vi "Scan and Trace(Unfold Normal Speed).vi"() -> ()   [LabVIEW 2020]
uses:
  Labview Library/Libraries/Basic Experiment/Basic Experiment.lvlib
  Labview Library/Libraries/LaoJi/NI CTR/NI DAQ Counter.lvlib
  Labview Library/Libraries/PIScanner_new/Library/PIScanner.lvlib
panel:
  in  "Stop Scan":bool
  in  "Stop ALL":bool=TRUE
  out "Laser On":bool
  out "Current Position":dbl[](array[numeric])=[149.3013306, 92.52485657, 114.2977448]
  in  "Tab Control":T1(tab)
  in  "md File Path":path=path "I:/Important Scan Image/Find SIV.md"
  in  "Comment":string="下午重新写了ASG的程序，把之前的Laser什么的用新的程序改掉了，然后把程序里面的计数都用老季的改掉了"
  in  "Title":string="扫描XZ"
  in  "Scan Parameter":T2={"horizontal start"=10.0, "horizontal end"=190.0, "horizontal num"=40, "vertical start"=100.0, "vertical end"=160.0, "vertical num"=40}
  out "Intensity Graph":dbl[][](graph)=[[17781.40531401807, 5714.199786500514, 6283.714545371459, 6735.417820419619, 5516.371803474795, 7255.943323026121, 6467.242901396061, 11976.047904166111, 11638.851498312759, 33572.80368126317, 34644.84074795653, 11401.592204703611, 12777.968493765737, 16629.229580655952, 14525.548166527793, 26871.089749350882, 27700.971050532404, 26252.009210884047, 25345.291111593357, 22513.920437453515, 23987.33624029484, 23198.350772809936, 23001.433789688253, 23079.35827112529, 24582.896751616194, 22567.526269993323, 24264.76234359153, 22164.571946750242, 25398.356910744176, 21846.320324133354, 22342.246318034588, 24552.890412679728, 24617.940704268913, 21673.961690578664, 26341.4103776154, 23416.335588634272, 24165.213215005195, 21944.877795249304, 24289.577304311242, 23535.77278446977, 25519.2278536345], [12532.419773169353, 6756.365461451473, 5205.122244571681, 6640.994524713253, 5430.964469504035, 7784.6001147647185, 6877.126979041758, 12219.704514135643, 12149.51945578161, 31845.833503515085, 35459.51140053275, 12611.918262761195, 10461.664756189162, 15261.448655811466, 13971.079864781508, 29604.672953223595, 26585.433397884048, 26165.899763849535, 22610.420936584742, 24458.55473918764, 21202.20584482011, 22676.314716648474, 22852.49041256598, 21138.005322471614, 23202.639601690946, 23660.949017499315, 22138.91430764288, 23771.110418104054, 22131.508001735023, 23840.890321990857, 22513.23380272118, 22045.969737474737, 22009.927882442946, 26290.801792700036, 22550.881393922507, 23976.253997987915, 23209.151892740247, 21374.168364274912, 22886.1538768692, 22109.997236054605, 22247.049582562136], [11023.148612036859, 6069.880132632881, 6091.825744562944, 6785.714285685821, 6272.541947646212, 7394.588598920568, 6863.383847160945, 12491.059826098322, 11518.116836241139, 33022.96459391927, 32198.322866861687, 12239.159240629258, 10380.206400641651, 15867.913649992137, 15146.431954406176, 29088.75642993861, 28241.281926540338, 25375.18296954822, 24239.543726400287, 22402.275786833994, 23427.467970935504, 19542.00015163378, 22868.559027272375, 23480.382191633205, 20472.903807809227, 23607.132086915753, 22000.15103086426, 21024.698918047514, 23190.641721682656, 21132.816105685317, 23244.46434584329, 20836.027647314855, 20762.358720963322, 24523.97567534188, 23514.537347734593, 22355.4414949403, 22273.56939147543, 22333.351986807338, 21172.97292010603, 23223.122196765806, 24603.867748041343], [12734.597431764863, 6547.24759851939, 6416.618185537506, 5721.2403649376465, 5517.269052163687, 6015.6693864512035, 6753.645433656194, 12558.695509637037, 10756.152568869344, 31460.58872169549, 29049.138481258386, 11605.03335797576, 12437.873324350952, 17971.080543714357, 17242.00048384432, 28463.531419469364, 27475.425557442424, 26130.076311780726, 23883.4365556246, 23337.802274226877, 23996.129656380228, 22192.4179121422, 22839.91858432976, 21200.737241837916, 20902.390142804205, 24376.990912244193, 20471.9645018656, 24101.790691422255, 20445.865161215617, 22588.842725292176, 21766.153377964467, 24164.48230671008, 21458.55170514228, 24138.01737736392, 24437.465471435327, 22589.395355642413, 21022.36718033937, 23901.075548187724, 21333.252640294686, 23447.659501746144, 21647.470177122526], [13703.182922298633, 5847.981715258857, 6706.874546456047, 6398.55097428461, 6057.052589773717, 6495.037310448332, 7086.934661307756, 13978.25044774562, 13984.747570265346, 34137.82564325823, 32511.9610057858, 13027.2184658737, 13741.34295395774, 17104.746207888747, 17614.610856088933, 28716.700446135794, 25474.792952360327, 25993.334782884132, 26240.48163660691, 22965.466183809942, 23424.85447434729, 24130.717249332658, 23824.887079750475, 21671.91895887727, 21540.144773083164, 22493.36115814037, 21465.475127230937, 21198.15668224017, 22004.76852760417, 23441.069548457646, 22470.987800033847, 22425.468296537474, 22085.716729267533, 21966.897808341815, 21877.303983712707, 22933.978416931946, 21511.349004124007, 23042.548454102853, 23403.759476785068, 23031.02748277378, 21486.356423589263], [12946.458625764166, 5592.979573231455, 5355.55804911163, 6146.06995703598, 5811.338679804044, 6541.940535257157, 7146.4081531214715, 15118.615175448802, 14260.249554349572, 38472.66562819246, 28917.599545080768, 14560.161779681965, 11942.44038600165, 16361.727963159978, 16676.65922683603, 25432.611286917556, 27901.729504499723, 23724.058258230565, 24343.84948213968, 20859.21325040204, 22430.7095897709, 23433.51497685545, 22768.02231275929, 22997.335154221877, 22810.76548338465, 22314.50442798871, 24192.1060310366, 21689.561203437006, 24769.464919970418, 22259.404975464142, 23686.52012581378, 23019.915940346265, 22912.675054829342, 22043.95615522176, 20784.300237402647, 21349.858766401016, 21467.934199254676, 22871.611588918604, 21936.194721343476, 23331.20947496009, 21118.625610036048], [15108.656825916609, 6239.1192779141975, 6312.801697329427, 6187.145950708841, 6446.4557386773895, 6470.551852386961, 7216.682142987088, 12868.087143887658, 13752.530847681093, 36714.44752569549, 28113.03868578447, 12293.244257602446, 13836.343120908285, 18794.407517710853, 18768.975986861362, 25842.66260191859, 25406.167741787198, 22824.072248460976, 25795.399654439527, 22353.416086401263, 23948.948576778093, 21186.880751003624, 23624.96134324281, 23580.111395671436, 24534.746642358583, 20651.686897780863, 22050.88587261794, 19474.63997207082, 22674.91145848678, 22042.50085991519, 22669.283121507186, 22841.203104769444, 21777.28499900127, 22078.463462280237, 22662.45054698885, 21249.18592330017, 24710.44891537157, 24516.148680604256, 23315.182906237365, 22286.48875660515, 22633.228531474746], [17795.150050280685, 6449.597404012824, 6894.2808339333, 6528.867983310664, 5874.048043502244, 6908.497960464559, 7213.827464483127, 16651.09660053513, 12867.285305575791, 35971.57415907753, 29429.045855353244, 12551.307710516148, 10945.904448630308, 16281.960409533162, 19222.490313605766, 26654.070650398757, 26805.763239121476, 24811.29438082978, 22899.081162413582, 23731.187617414285, 23128.12605779083, 22971.692787986452, 24516.263780919406, 21873.533024952452, 23038.317695560658, 22377.149974604214, 23126.1531654435, 22219.3882555528, 22362.94631813883, 21501.638692924065, 22635.58251984891, 22797.809337764254, 22281.266483187715, 23329.044660590105, 23010.873002359025, 22861.62499276789, 24632.17821041294, 21650.54102304532, 20874.01857241737, 22453.997957870415, 23459.415211780753], [21338.133570599763, 6555.311072382466, 6775.513093407144, 6111.9754308429065, 6544.272000090105, 6510.252385821501, 7185.775222879924, 12227.57341226559, 16303.87562026553, 30869.41392847601, 27481.140393748512, 11543.097636165548, 12221.454691293859, 18336.659100022796, 19224.188256100613, 28038.05753978185, 24342.319018456106, 24396.416459955657, 23920.702869922625, 23977.903906220236, 21903.03066421081, 22772.864979987382, 21670.825470269407, 24525.1752708809, 22664.204382525186, 22220.00299592514, 23771.790808245398, 22157.446392871057, 21293.69643948261, 21261.329703702413, 21582.11996661651, 23605.76923101778, 22359.89890311861, 23960.920511407538, 22528.505455925613, 23643.49635986227, 22556.50480143065, 24655.407702004413, 22511.657822725963, 22889.11495408441, 23631.332198683845], [23701.73240945884, 6492.206911036676, 5922.018462721852, 6323.840880128348, 5629.00381575497, 6997.596687497127, 6702.179946025261, 12335.56641207772, 17603.66318997689, 29868.977297675126, 24782.897785669807, 13519.914735665314, 11702.457516175964, 20474.271160404962, 19056.03295513057, 27380.034884381206, 26013.15002973438, 22466.071646735894, 23673.748232861275, 22622.066979178308, 22917.517354168216, 22937.991301636022, 22038.59441653508, 22228.549449716407, 24077.168850077833, 23535.365108564783, 24152.001791906245, 23546.932861186102, 21065.807751551467, 24501.13790840757, 23818.33768449075, 23703.837908006444, 23741.810338232306, 21583.138556603993, 21670.879077564827, 22826.997978787636, 21502.856007388713, 22849.635119916536, 22203.058867879732, 24580.02909866139, 22143.665719878663], [28910.63890969335, 5374.048868646638, 5433.751800549745, 6801.336703616646, 6151.568890369337, 6693.337829650435, 8132.216710997627, 16889.924286506568, 13870.41219359557, 34905.62174980876, 25513.72224539108, 12485.352736778397, 13535.027970696072, 17102.10875102997, 19732.098812215376, 28482.075934825476, 28048.0678843836, 27727.455716477867, 24103.84114433336, 23653.07560931371, 21217.29209304353, 24687.029814389018, 21563.838653968593, 21448.791649757946, 23713.982186983216, 21326.573212064995, 20203.360083890242, 20296.206962447108, 22585.545251147654, 21959.27186084977, 20847.179653890533, 23326.69975051675, 22967.166521568648, 23572.751532103957, 21801.82144303294, 21422.877640464976, 21769.669917903808, 20914.87341946959, 21004.84803838279, 22930.47439936271, 22464.14377055246], [32647.49758123644, 5419.267431169652, 5810.488677035144, 7134.594117990506, 5868.883372794403, 6609.555972125465, 8172.94754364124, 14441.809037176925, 16817.48253758604, 30383.02535254297, 22961.83733052953, 12589.108090175867, 11015.960681427541, 16201.687597892624, 21271.215434178175, 27422.487446030267, 25342.655930594094, 25557.92012099764, 22001.928258963715, 23873.079828750277, 20357.896853300033, 22297.206903328253, 23011.51058968109, 23582.101383041612, 22051.350884986514, 22721.27079676657, 22958.99101284016, 22595.238931890857, 21289.24340243472, 23368.66856649395, 22798.84295867806, 23143.140323070907, 22480.759261516447, 21430.753369838214, 21976.836022512973, 25055.825718472326, 22307.614812332096, 23216.6695686924, 21879.342168171945, 20569.301951268702, 21815.36043207429], [42424.33718498176, 5961.643392651804, 6350.043717628025, 7344.770189793268, 5874.054252150575, 6623.955950636146, 7995.518435530115, 13587.85878848428, 20864.30766158807, 30510.72297139569, 23657.23715889375, 12156.41923702506, 12708.796161785125, 17646.09932229004, 19430.475643868776, 27398.372333622145, 26190.55855062135, 25611.098772989655, 22057.35934602098, 23833.320519690875, 22573.13544381975, 23404.011118143902, 23295.36870525358, 22449.323204105003, 22418.188015336433, 22170.46852913932, 21997.51822867481, 21145.233374717267, 22745.36563167298, 21942.948334494315, 22337.479536644052, 22001.320079021316, 24019.256376062633, 22316.401531370215, 22586.366323655613, 22802.89937317404, 22402.518769645092, 22787.088284472946, 23505.708529067895, 23583.500486684094, 20603.586986279242], [29689.38757970999, 6943.6187667738795, 5853.866212559558, 6179.21809527893, 6251.6013323226525, 7254.622337249093, 8233.799237608442, 13149.243918481287, 18449.244192560134, 29332.94885616236, 22384.74157892232, 12006.430222048573, 10548.523206727543, 18099.03027291847, 20293.232352592917, 27573.244658312044, 26197.973677519258, 24158.21379291054, 23786.251161511864, 24268.31530745387, 21437.793856159755, 22572.12616456447, 22086.729297467704, 24425.96423682751, 21378.40780826053, 23436.064727228626, 20909.858667660454, 21441.684004543524, 23680.78112543714, 22367.805785739645, 23814.47007750817, 20998.517454045155, 23014.36054452742, 21627.659034424516, 23580.412811549075, 22096.734593853253, 22821.437798471943, 21818.628806914276, 21628.28656483592, 23831.569999409214, 23568.230025772962], [23911.102291849384, 6186.718172367911, 5836.859769492626, 5293.352557479528, 6348.221771021702, 7506.313256842828, 7701.594438161941, 11811.35577496218, 22098.54313321218, 28979.38237691486, 22408.325262608418, 11336.192025335593, 12700.140608740185, 17440.536568355274, 20830.780541491215, 27567.0511087282, 26303.854875240915, 22258.021466782764, 24306.82417878424, 21437.129305794893, 24228.695951306825, 21797.939860690156, 23190.13953315866, 24199.462234073668, 21762.47129247648, 24181.57532786255, 21368.70037179639, 24864.558906915747, 23310.662571433477, 23059.657897322726, 21817.487408359677, 24075.97965606493, 21639.341015166174, 22892.16211140045, 23832.819046065393, 23498.810280425558, 19686.841864293634, 22182.595267963174, 23897.735358218793, 22374.65626225276, 20779.6440976457], [20983.947280497385, 6947.451570091462, 5543.210761451669, 6456.6503498567745, 6374.829704705129, 7469.94404595482, 8093.065285732568, 12671.212212668606, 21672.013435625246, 25146.731430728058, 19265.966669958543, 13123.426593051756, 11901.049786877067, 17357.34432642321, 21458.67532544291, 28969.375232126597, 25038.853393407735, 25099.455351896548, 23475.100677497016, 23386.27314575218, 23286.304130815723, 23019.26645972914, 22710.944167757007, 21492.903930234923, 23069.581327771943, 22747.562581042534, 21600.011368559095, 23793.171114690966, 20602.120258433533, 22950.788121448884, 22533.627864879058, 21731.36764785229, 21550.313436163586, 23192.641117184783, 22115.758125117514, 23449.36578974685, 22371.903974204153, 23323.979445834862, 21624.523323570775, 24683.4186060647, 23853.383180259658], [15158.598608774711, 5581.107949583157, 6355.771419891991, 5759.243585960283, 6748.414122656793, 7827.1597258861675, 8666.673544993906, 14166.805309843918, 26003.985561439917, 26307.598076273032, 18802.18126148224, 11989.184225315421, 12213.801595793395, 17208.934995988624, 21055.969243440006, 27328.24427487038, 25444.271024030408, 23833.129957485544, 23236.207357609706, 22836.507896161034, 22503.949368399863, 22868.42724564458, 20564.2965127695, 21603.858266644744, 23224.33787585145, 22996.2420775463, 21882.153780969074, 22329.216384033167, 21503.269041127176, 22563.199724799906, 23172.379665395663, 21750.35206518319, 20402.869371726494, 22046.166081296346, 22291.340195545636, 22497.964822087357, 21944.238860866022, 21953.55899006688, 21539.783877163893, 22363.329885570212, 22256.15279102048], [13906.55822985576, 5593.602128592306, 6179.000903092564, 5629.665891541231, 6348.566533976336, 8021.444672294558, 6659.530281141814, 12866.895747871224, 25358.4021176122, 25792.60486469167, 18737.568825491857, 11550.678602384663, 10954.911369241214, 20075.740292802904, 21440.470559141202, 26447.966604056157, 25815.330109146264, 23270.04282894463, 22715.726121595115, 23041.818661247307, 21928.731622054253, 21474.803397844797, 21328.443317804064, 22684.01930050322, 22676.19301422577, 20753.29395262562, 23246.52944478169, 22508.918384714827, 23672.0669609167, 23544.33591261006, 20815.229472887786, 22034.829886086864, 22545.791367463873, 21965.446848819476, 22990.46321522983, 22172.08839716104, 23075.511957728057, 23338.007337504074, 21794.125375565633, 21480.151374786114, 22756.93746936868], [12716.909436486196, 5575.535954650932, 5482.483971341909, 5934.980085920285, 7535.866910818768, 7559.166006571037, 8452.657525603563, 15944.115873773313, 25264.25388800804, 27943.330724664298, 18457.5797312275, 13109.728426951648, 11319.642940302838, 19347.871734198197, 24349.39845686028, 26087.220295553365, 24774.030809819218, 24318.721876773183, 22954.058478102157, 22194.598044588765, 23885.883873561463, 20845.206372463595, 21616.088332975236, 20693.846836680576, 22551.88695867547, 21710.54004957192, 21442.504802121446, 21019.871942016438, 22946.05970860647, 22332.16692907884, 21117.156222869937, 23272.654630832832, 20473.822755307672, 21017.577028334905, 22291.05311254134, 23417.029441410785, 22176.51702944195, 24064.666076864105, 22839.194237198397, 22807.093197714818, 21741.531849294402], [11726.766344090087, 6255.455338957476, 4853.968361824107, 6926.762622225452, 7062.111521238783, 7945.743388378028, 8335.620546227106, 16764.33350509733, 29800.989999276262, 28566.776690697287, 19903.698268117856, 10639.607910766705, 12518.255789754128, 19128.797264389683, 25434.76286124696, 27012.20206384351, 23481.168688444974, 23006.912209109487, 22430.89754191115, 22439.122560051685, 23825.486050178548, 24330.65562062395, 21289.429798034285, 22347.817845115333, 22552.501117636228, 22582.97113810702, 22863.549944008028, 22079.645141412486, 21681.620383853187, 21102.277976465455, 22898.53025734539, 24737.835516611107, 23126.638997431342, 22709.778591587146, 23677.310656248115, 22733.05116447157, 21881.838074406496, 24941.378131560443, 23302.10953529628, 24069.394878566163, 23460.530207933887], [12570.482644479478, 5906.85045736545, 5616.887427308557, 5969.822547048601, 6143.614298035342, 7820.606531510265, 8086.331212310732, 13762.336220475165, 30665.748370020025, 23184.88041733266, 16572.296644113838, 12168.983614429317, 12461.6564416735, 20693.249934729723, 24522.656466912027, 26845.442100206674, 24849.680571315206, 24302.246086430878, 24013.11640822098, 23474.987081474257, 23038.44128507233, 20589.68868403232, 22067.543697378263, 22154.709515883438, 21238.938052969374, 23016.147427256652, 23105.33777458174, 21886.3108354753, 22456.249032066953, 21740.49049053781, 21833.539565424657, 24691.972619732973, 21707.16684216407, 22357.090463144672, 21654.209931401223, 22658.82554125862, 22963.471508667393, 22166.610664988475, 21617.491064012287, 23349.99268729444, 20848.99513858946], [12453.491589986803, 6154.722605080047, 6226.532576073008, 7327.23747880051, 7068.625829055126, 7642.199497801821, 8211.189835869827, 18918.659852618388, 31289.78327199429, 24731.35312189666, 17212.15146702176, 11456.4890121429, 12306.202527852223, 19791.837607417787, 22693.993388260304, 25842.280280488783, 26060.01916477979, 23957.35590645255, 23817.349509885553, 21501.923984423887, 21714.198333229513, 22397.73063538625, 22792.258920211796, 21837.054445698584, 21759.542155304276, 22899.685255307428, 22557.43083748549, 22060.96383944774, 23205.853144645076, 22101.187875301133, 21272.59594933882, 22653.705133802578, 21815.825837915345, 22495.47810480767, 22911.843952860658, 23068.165434619612, 21828.186788411167, 22586.380892775072, 25134.29853149532, 22844.911861836445, 21243.7913387969], [11155.789358839924, 5739.956262483621, 6826.516782272394, 5627.247322285265, 6446.653938633454, 8029.045957455128, 7729.10741440906, 13266.795252422751, 37795.4190132485, 29436.218943624717, 18266.61291216888, 12282.135466683621, 12017.439708393023, 21625.02516043149, 23767.082590557107, 25646.959003469696, 24780.532806028474, 21811.572250814508, 24630.54187167741, 23566.944530424036, 22840.345981674393, 18712.593880717857, 22789.516822257137, 23071.16410089152, 21680.68684420017, 24975.45255427038, 21551.832408074413, 22642.31767584701, 21936.17813816276, 23633.468236997727, 22212.7871091394, 23028.730604113272, 22191.098956352114, 23264.50295155943, 21580.59622896799, 20944.961020516337, 21851.196430003485, 24954.559604587037, 22583.490092182645, 25107.56718472896, 22805.071390793953], [11130.45609339241, 6225.05039326186, 6031.518550789189, 6256.161371053009, 5526.759974349571, 6995.435095619068, 8622.158948439583, 15303.93617236037, 34729.799375124356, 26661.8645297555, 15833.61425235118, 11895.605804243749, 12191.704724766858, 19996.699573830294, 22384.65957484329, 24393.486887785555, 25321.302922442064, 25235.895537827957, 22786.194604357843, 23918.872144849058, 23020.71369165517, 22993.72210875554, 20349.88030917671, 23270.315898494384, 21091.643189722905, 22271.82714654106, 21819.445366908276, 23223.760936728417, 23936.8898695451, 24597.714666568754, 22519.789750692453, 23938.400548968726, 22853.458126501253, 23600.12715182123, 23453.458754805513, 22384.789773422926, 22124.11329935702, 24296.719942989996, 23466.9050606385, 23937.36133053921, 21615.061334644688], [8876.034706260767, 6996.446008220829, 6725.391640310086, 6574.939810335698, 5366.708182737018, 8628.127696203717, 9318.684679645916, 14019.123522397747, 38248.66129669711, 24315.952503896082, 16567.01356976382, 14070.179775021532, 11726.005790379391, 22572.128889784988, 26887.487307066087, 28341.3181919563, 26491.145843873936, 23801.09843779488, 23686.88955851646, 23448.199538002656, 21661.990427588575, 24187.306501426112, 19558.19700711089, 23172.939314538795, 22273.605777253513, 22214.393361060214, 23789.958507122625, 24431.064001609426, 23970.50717359679, 21939.65051049769, 22873.13290291404, 23960.943661924222, 23738.473393705433, 23648.15569549645, 21407.990973393637, 23514.193749088383, 22212.81997052337, 24511.50996890828, 25257.02739667838, 24461.315063735507, 24266.10146444408], [8518.322043570464, 5984.174085032187, 6935.5240472430205, 6273.460669072998, 6469.902605757591, 8818.11740843145, 10495.371337446079, 14445.041655434396, 39294.76497101231, 24997.849375445963, 15514.688417690057, 12575.333364900816, 14171.34638367847, 17966.865526454207, 27087.781823023433, 25211.8896979266, 25165.737991857583, 23193.586119897253, 23629.74498545509, 21651.377973390667, 22290.53813606203, 22129.246899706777, 23686.066682981007, 23618.866087044637, 22667.345145152343, 22011.350553602904, 21385.64774136008, 23150.18163597523, 24170.703174096627, 21869.954498863, 23082.89119232677, 21761.67391189705, 22978.56507144082, 24767.486304027443, 22096.770285512266, 21794.048826772112, 23153.21494059085, 24428.77622087736, 22048.565379833868, 21396.80372510928, 23525.392293173525], [8366.05332718353, 6215.583633644127, 6147.540983618353, 6368.666162536263, 6543.689876848047, 6824.617022796105, 10786.107901913872, 16064.410636925859, 39970.614107181165, 24437.460716413363, 15342.114103146927, 10531.428133160323, 13233.003403403753, 21880.59593674227, 27125.73846497478, 27169.171714301516, 27216.013551331274, 22746.275167655956, 21803.857842853595, 23306.510754137158, 21133.477235006867, 23672.140849183303, 23187.642707703413, 24321.832767852076, 23098.16721054929, 25123.16541581317, 21539.262172002327, 21223.734371357332, 21112.30862356185, 22356.829320686087, 22730.62430384153, 21699.856718673527, 21766.84598410826, 22973.981965373678, 23794.416243708132, 23342.15468253403, 21828.089864639936, 22699.319020425944, 24037.496487233104, 23639.950009675278, 22940.32971010913], [8077.627018081368, 6695.480550626798, 6173.945948072265, 7288.593351394921, 6366.369401043135, 8184.576307046574, 9290.786553010501, 15986.733989629574, 40151.87470335294, 25733.008570819147, 14065.162292060648, 12648.005993091547, 13932.657135019279, 19574.12647366205, 23720.77261945688, 27408.21950278449, 25418.932303578356, 24099.397515154054, 22187.242335646333, 22581.16200340387, 24966.12087681414, 22659.234025016212, 20979.56184617982, 24019.956539905084, 21644.687797286642, 25665.604997229395, 21674.058443606897, 21205.362711539816, 23501.593205957703, 23678.539019847383, 20706.9247807979, 23415.141791736183, 20438.310702721832, 22898.553721176555, 21778.60290525198, 23358.434935200217, 22416.455409961152, 21530.119946329272, 23844.945648979585, 21264.489748563243, 23398.536582676745], [9052.056746016631, 6526.309496511795, 5448.054709950722, 7265.975053540961, 7251.808085039935, 7601.079252576243, 10047.661986375018, 14382.25269415205, 33310.99459955877, 25094.29142443203, 14578.232235425707, 12190.586387976735, 12617.097872629185, 20757.965120578843, 26479.332700021518, 25941.782990727083, 23780.44220654035, 24347.497037559056, 22422.685750880282, 21513.924427928454, 22647.032645265015, 20282.253028605577, 22327.239231661864, 24250.342721602887, 21789.63472727316, 20879.12614141989, 22528.087438059312, 22564.04347676142, 21153.827055029204, 23964.119406775775, 22891.443686858536, 24015.84550624457, 21890.077669664457, 22824.60463652431, 20528.307845563435, 23549.96025960598, 22637.152276684537, 25091.770828470202, 23131.72593649845, 23516.392308669063, 21169.94478498504], [8254.692945777426, 6608.3957602643795, 5483.363681474447, 5918.706565304035, 6537.284980739362, 9111.61731205816, 10993.738349004207, 15441.674521789593, 35904.83056977817, 23450.958063258513, 13453.457084933, 12713.971526743919, 12621.92212373219, 19426.16531557143, 25573.655631349848, 24758.666809507708, 25220.501949520527, 22613.761063214293, 22086.614785646187, 21978.553965971965, 21215.015623343166, 21934.92803063654, 21775.80727424962, 22288.153288115656, 20315.862040154854, 20821.248031868214, 20734.223576490513, 21617.862703872357, 21992.81636510743, 23567.396276188174, 22145.386552137174, 22608.713688652402, 22363.17801096763, 20980.03884827361, 23013.4019223794, 22297.12457045188, 21384.440802140805, 22334.31972325313, 21483.808234018314, 21714.42487226501, 23346.855264772872], [8345.21533044442, 7336.302296953754, 5026.87841111217, 7253.2387726115785, 6508.1503231779725, 7455.960285250554, 10946.529654222115, 15515.75143369043, 34939.64541663416, 25074.471179208525, 11938.87297036689, 11349.592675779155, 12683.11243574654, 19066.384346971077, 24747.687653334255, 25703.959956111623, 23766.171538284685, 23138.194401816345, 23585.36160997812, 22743.322394234794, 23578.302067549197, 21152.12670828942, 22736.26942481772, 21231.823200304887, 22529.58232116407, 24477.681963460185, 23042.53652242069, 21953.48311330797, 21885.6900889559, 23234.753809883718, 22117.43516903794, 24206.403872886793, 21687.1145173245, 20839.185841527185, 23019.634394083507, 21468.208832412627, 21280.90272565855, 25173.784935832144, 21050.151602065893, 22048.457827589566, 23687.66529039607], [8133.346211139868, 5669.588428029329, 5350.693360685931, 7390.023468307687, 7052.149876223108, 7344.2798075534165, 11516.410885448073, 17257.996962168414, 36041.59189603943, 25328.1853282432, 13794.915588269996, 12484.27643210644, 14205.158968226448, 17431.459196605043, 24508.418667406197, 26484.26279798435, 23479.445050234757, 23885.267815568503, 25549.519474295554, 23763.035614456243, 23802.409092377326, 22851.633120298437, 24324.74507668369, 22669.62828920628, 22846.96603498021, 22287.650900768498, 22360.03059280616, 24977.931145397153, 22282.54455339705, 21642.72849713222, 20999.099327682048, 23697.042427023778, 22535.606257971915, 22893.00052531996, 22343.22819168509, 23046.27021003501, 24239.930140810306, 24195.79357650442, 21760.812403597978, 22482.43077776127, 23188.104398344378], [9113.658907518624, 6556.335827809229, 6595.833887237049, 6495.728190970752, 7226.601980975829, 8746.894852358124, 12964.249784767057, 18172.403835648285, 37621.55428766609, 25263.48023588519, 13860.566687861563, 11550.417572791985, 13953.862381791165, 20399.816451627867, 25881.379532993953, 26299.062064814127, 23116.232105500487, 24480.04776599344, 22583.377021330198, 20512.37708179464, 24257.473020602745, 24550.618041732792, 23654.135186461088, 23085.860287720552, 21138.26656510308, 24044.205495833954, 24403.274948389866, 22139.996029869333, 23747.586291640306, 23452.67692688313, 21082.742340188797, 21482.38805676368, 22037.55794130076, 23790.07555660264, 22891.566265110327, 23749.88125079115, 21529.14604247496, 25073.508680049756, 22823.790082757565, 21293.178541657762, 21327.136586757813], [7645.688596262476, 7435.0602083338845, 5544.085034801818, 7516.369786121573, 7403.463400963354, 7925.394324796851, 11682.831273704727, 14236.43432068073, 35532.81087325775, 25438.312093136126, 10526.845975556798, 11107.600088073576, 15611.308630463605, 19744.32601183629, 25693.681646689856, 27571.58006373659, 22446.35617511643, 22796.78078710177, 24787.797688181352, 24321.056990334186, 22328.713897054415, 23324.201372213545, 22385.65733104416, 19805.851214422222, 22135.090508561334, 22836.628356167876, 21163.043002515165, 22529.251294225185, 22401.56810975863, 22356.883580004916, 21803.558420676254, 23724.4961666394, 21622.880755298374, 24308.505616720995, 20590.970809471597, 23641.59344319865, 21268.368136159886, 22886.590515167103, 22899.144815990043, 25620.241438443347, 22297.320837480707], [6912.30967146747, 7117.4736502508795, 5700.873620346438, 7049.972469112892, 7704.902244062226, 7495.3345366723715, 12947.820785927604, 15601.306427201058, 35292.604501848815, 27656.82912897375, 11807.82760564356, 13018.706093669176, 15696.175797251284, 19688.449967721415, 26932.584987566563, 26645.54944603539, 20705.83904666913, 24669.08260572176, 22636.323214503915, 20063.04122270119, 23202.085714275625, 21851.132686005934, 21685.379595565762, 22586.136619581484, 21723.388848868937, 23030.675650606725, 22346.79735859369, 21601.38991262695, 20891.01179431534, 23123.678646851946, 20809.541936308877, 23744.063984175507, 22469.363318587635, 20649.530738254536, 24181.648596082385, 21896.851232804158, 22439.904092448167, 24697.271325748767, 21332.373804877327, 23003.89606464483, 24718.67555755913], [7702.676680184053, 7395.451797158753, 6057.492876424266, 5666.193617438352, 6457.005851333211, 8285.948067831805, 17152.131728376335, 17316.46352466374, 47099.045772369514, 28137.42693087479, 14100.888253011683, 11580.637935938634, 14000.267142875928, 20042.18904721772, 28095.622332411654, 27128.515595094424, 23173.384581794384, 24868.386608871842, 23033.62909873443, 23583.13053514905, 22442.33849177567, 23376.58566345161, 21137.22346753071, 21694.38165974286, 20361.261188548753, 22481.354147242364, 21489.015901781775, 24467.65306071732, 20877.2550770471, 24150.346886665244, 21526.437762349728, 24039.46218207583, 23212.556302018445, 21256.038647308626, 23063.480452130094, 24294.290841840582, 23185.363642744956, 24686.047250561875, 21893.301045228243, 23353.411671742433, 20779.6684828058], [6161.707243739151, 7529.930209237194, 5822.170027305326, 7029.304048014763, 7007.252506368001, 7761.346411217268, 13824.776811894264, 16340.968731064375, 36182.63332467868, 26078.01929794882, 12852.077998890152, 12272.197336898116, 15398.085806687568, 18466.70680433287, 27266.126283549253, 27038.60096390421, 24196.85440892928, 22179.46800217777, 22860.312966437225, 22197.784294687055, 20185.871913175797, 22882.757583711544, 20055.891799825837, 23607.44486858287, 23344.032681541546, 25371.330396718324, 20922.542698564117, 21207.610269429457, 20965.981004819852, 22057.110568050324, 21893.45851505012, 25737.3968461604, 23023.206172096827, 21602.315768122684, 21881.942848412316, 23830.71145226471, 23181.612973387477, 20839.221810859675, 22961.53691896497, 22186.241697904126, 23882.900527040616], [7088.127386643649, 6912.734034976467, 6536.147962091539, 6446.100876407494, 6986.083119269964, 8340.995042813063, 13745.088371847773, 16236.919567479012, 37333.13041878851, 26986.96652177176, 12286.607597721566, 11782.811523029559, 16102.246742923262, 18990.13539454356, 25568.19646258992, 27158.63928249937, 26571.11409588689, 24235.45872482386, 23431.48575822062, 25087.349151361068, 23379.467500416384, 22687.572998319865, 22541.19726539205, 22794.784553303227, 22943.813038566055, 23579.007538032856, 24363.11102840251, 24179.77663955669, 24216.148159936565, 23676.269568896067, 21743.967313251782, 23792.361240421746, 22422.75910046265, 24105.962999475996, 22114.31399238368, 21047.708138363374, 22062.736709463352, 24833.20023707679, 20847.71242447739, 22662.918900981822, 21215.679004725636], [7084.807195719434, 6815.221671383885, 7056.327001556509, 7643.948785591148, 6924.289523717523, 7388.422087846833, 14986.867439873577, 18599.507364482844, 36658.97826011614, 32460.354149418017, 11163.18310188526, 12168.032765564185, 16179.743165746237, 19205.519656142646, 26560.757106428828, 26779.92342599567, 22534.56951543325, 23113.33609189968, 25228.586281989366, 22384.884642922887, 21395.589523021543, 23047.144898751525, 22854.699230429083, 23737.43977633036, 21550.649013829032, 21863.69900639858, 22530.628343229087, 23077.212310563657, 20753.146780275263, 23793.073247767534, 21303.901437447734, 22537.885771202273, 21587.0600993252, 22620.207722270956, 20959.934858347566, 22805.01710368692, 23502.649947488, 22501.72799135012, 23987.261936536604, 22341.37622894133, 22976.574978796507], [6459.887399932155, 7328.691828520233, 8002.0130850195565, 7736.305450009826, 7190.892886086089, 7357.562194424906, 12411.868011952722, 11806.08261281461, 32049.002735461814, 26889.46509149266, 13854.71163575821, 12892.87594791113, 17034.919071556786, 19598.447457787435, 28354.46170337898, 27576.579918424428, 23306.833997808757, 24497.865390789382, 24750.629948253918, 24959.028101489755, 22963.048188849763, 25132.164753166668, 22031.470687619156, 24869.296336095304, 20705.41196637979, 23890.970299046734, 21342.334155419318, 23784.24089851782, 21630.13419224704, 24549.84089822509, 23350.172239018815, 23358.065402610224, 21382.930974494117, 24057.450628358525, 22849.504150110923, 22999.5450637245, 21882.476512795743, 24560.99636405485, 21828.498928641835, 22772.9874248827, 23049.98106767945], [8312.84159797885, 6996.326928398113, 5514.807257450751, 7293.090434247198, 6256.056144587044, 7769.6256810895575, 14716.52115317322, 12237.273235766766, 31894.621384065864, 30210.570688881766, 13290.239172666123, 13062.147797447686, 18727.488441641748, 19696.732843659687, 28496.534741899315, 30352.521420037014, 25367.376652972067, 25666.899531631014, 22995.261738618887, 25864.131846049328, 22891.676586332203, 24669.08260572176, 21619.557702057846, 25865.336351838683, 22197.22831921782, 24129.975004808777, 23862.306792173622, 23293.208902386297, 24394.10582987501, 24089.37566684125, 21916.62654474708, 24831.729101125475, 22520.817562620858, 23646.655582725143, 23226.046204167415, 26639.669074855094, 22194.575765275138, 23881.242414405708, 22125.406609452257, 24121.08161837743, 24250.356056702803]]
  in  "go to crusor":bool caption="X"
  in  "Horizontal axis":i8(ring)=1 items=["x", "y", "z", ""]
  in  "Vertical axis":i8(ring)=2 items=["x", "y", "z", ""]
  in  "Save Scan":bool
  in  "Start Scan":bool
  in  "Path":path=path "I:/Trace/Trace Stability.tdms"
  out "Waveform Chart":dbl(graph)=13702.436734038685
  in  "Save trace data?":bool
  in  "-1um":bool caption="X"
  in  "Tracing axis":enum16{"x", "y", "z"}(ring)=enum."z"
  in  "-0.1um":bool caption="X"
  in  "+0.1um":bool caption="X"
  in  "+1um":bool caption="X"
  in  "-5um":bool caption="X"
  in  "+5um":bool caption="X"
  out "counts rate":dbl=13702.436734038685 format="%#.1f"
  in  "set trace data save rate(ms)":u32
  in  "milliseconds to wait":u32
  in  "Tracing":bool
  in  "Goto cursor":bool
  # "The program will\natuo save your data\nBut recommend use\nthe to save comment"
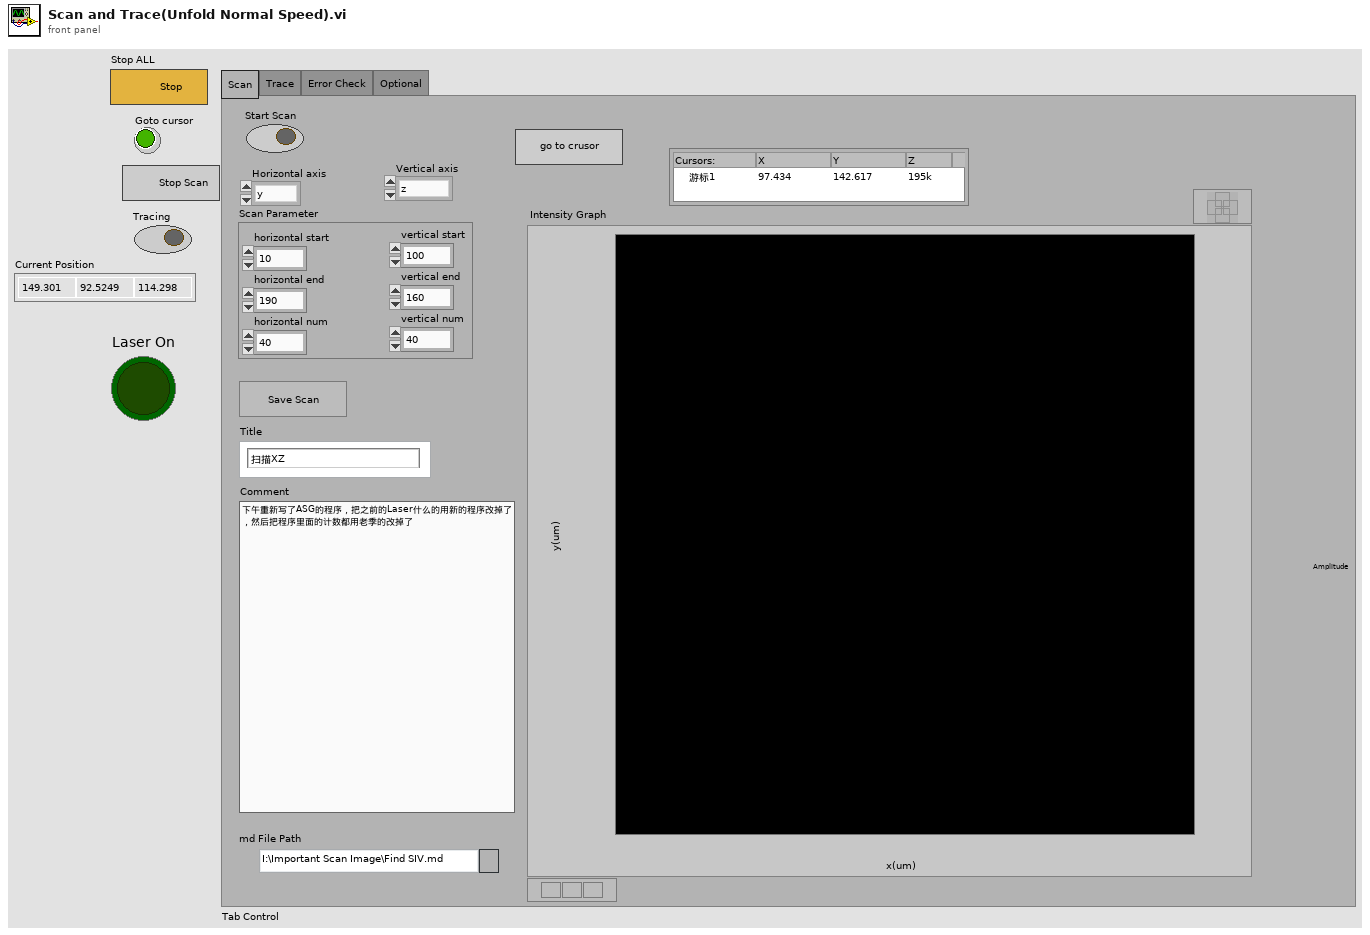
[diagram p1: front panel]
types:
  T1 = enum32{"Scan", "Trace", "Error Check", "Optional"}
  T2 = cluster{"horizontal start":dbl, "horizontal end":dbl, "horizontal num":u32, "vertical start":dbl, "vertical end":dbl, "vertical num":u32}
  T3 = cluster{"Horizontal axis":i8, "Vertical axis":i8, "Scan Parameter":cluster{"horizontal start":dbl, "horizontal end":dbl, "horizontal num":u32, "vertical start":dbl, "vertical end":dbl, "vertical num":u32}}
  T4 = cluster{"Horizontal axis":i8, "horizontal start":dbl, "Vertical axis":i8, "vertical start":dbl}
  T5 = cluster{"Title":string, cluster{"Horizontal axis":i8, "horizontal start":dbl, "Vertical axis":i8, "vertical start":dbl}, cluster{i32, "position out":dbl}, "Comment":string, "md File Path":path, "Intensity Graph":refnum<vi>}
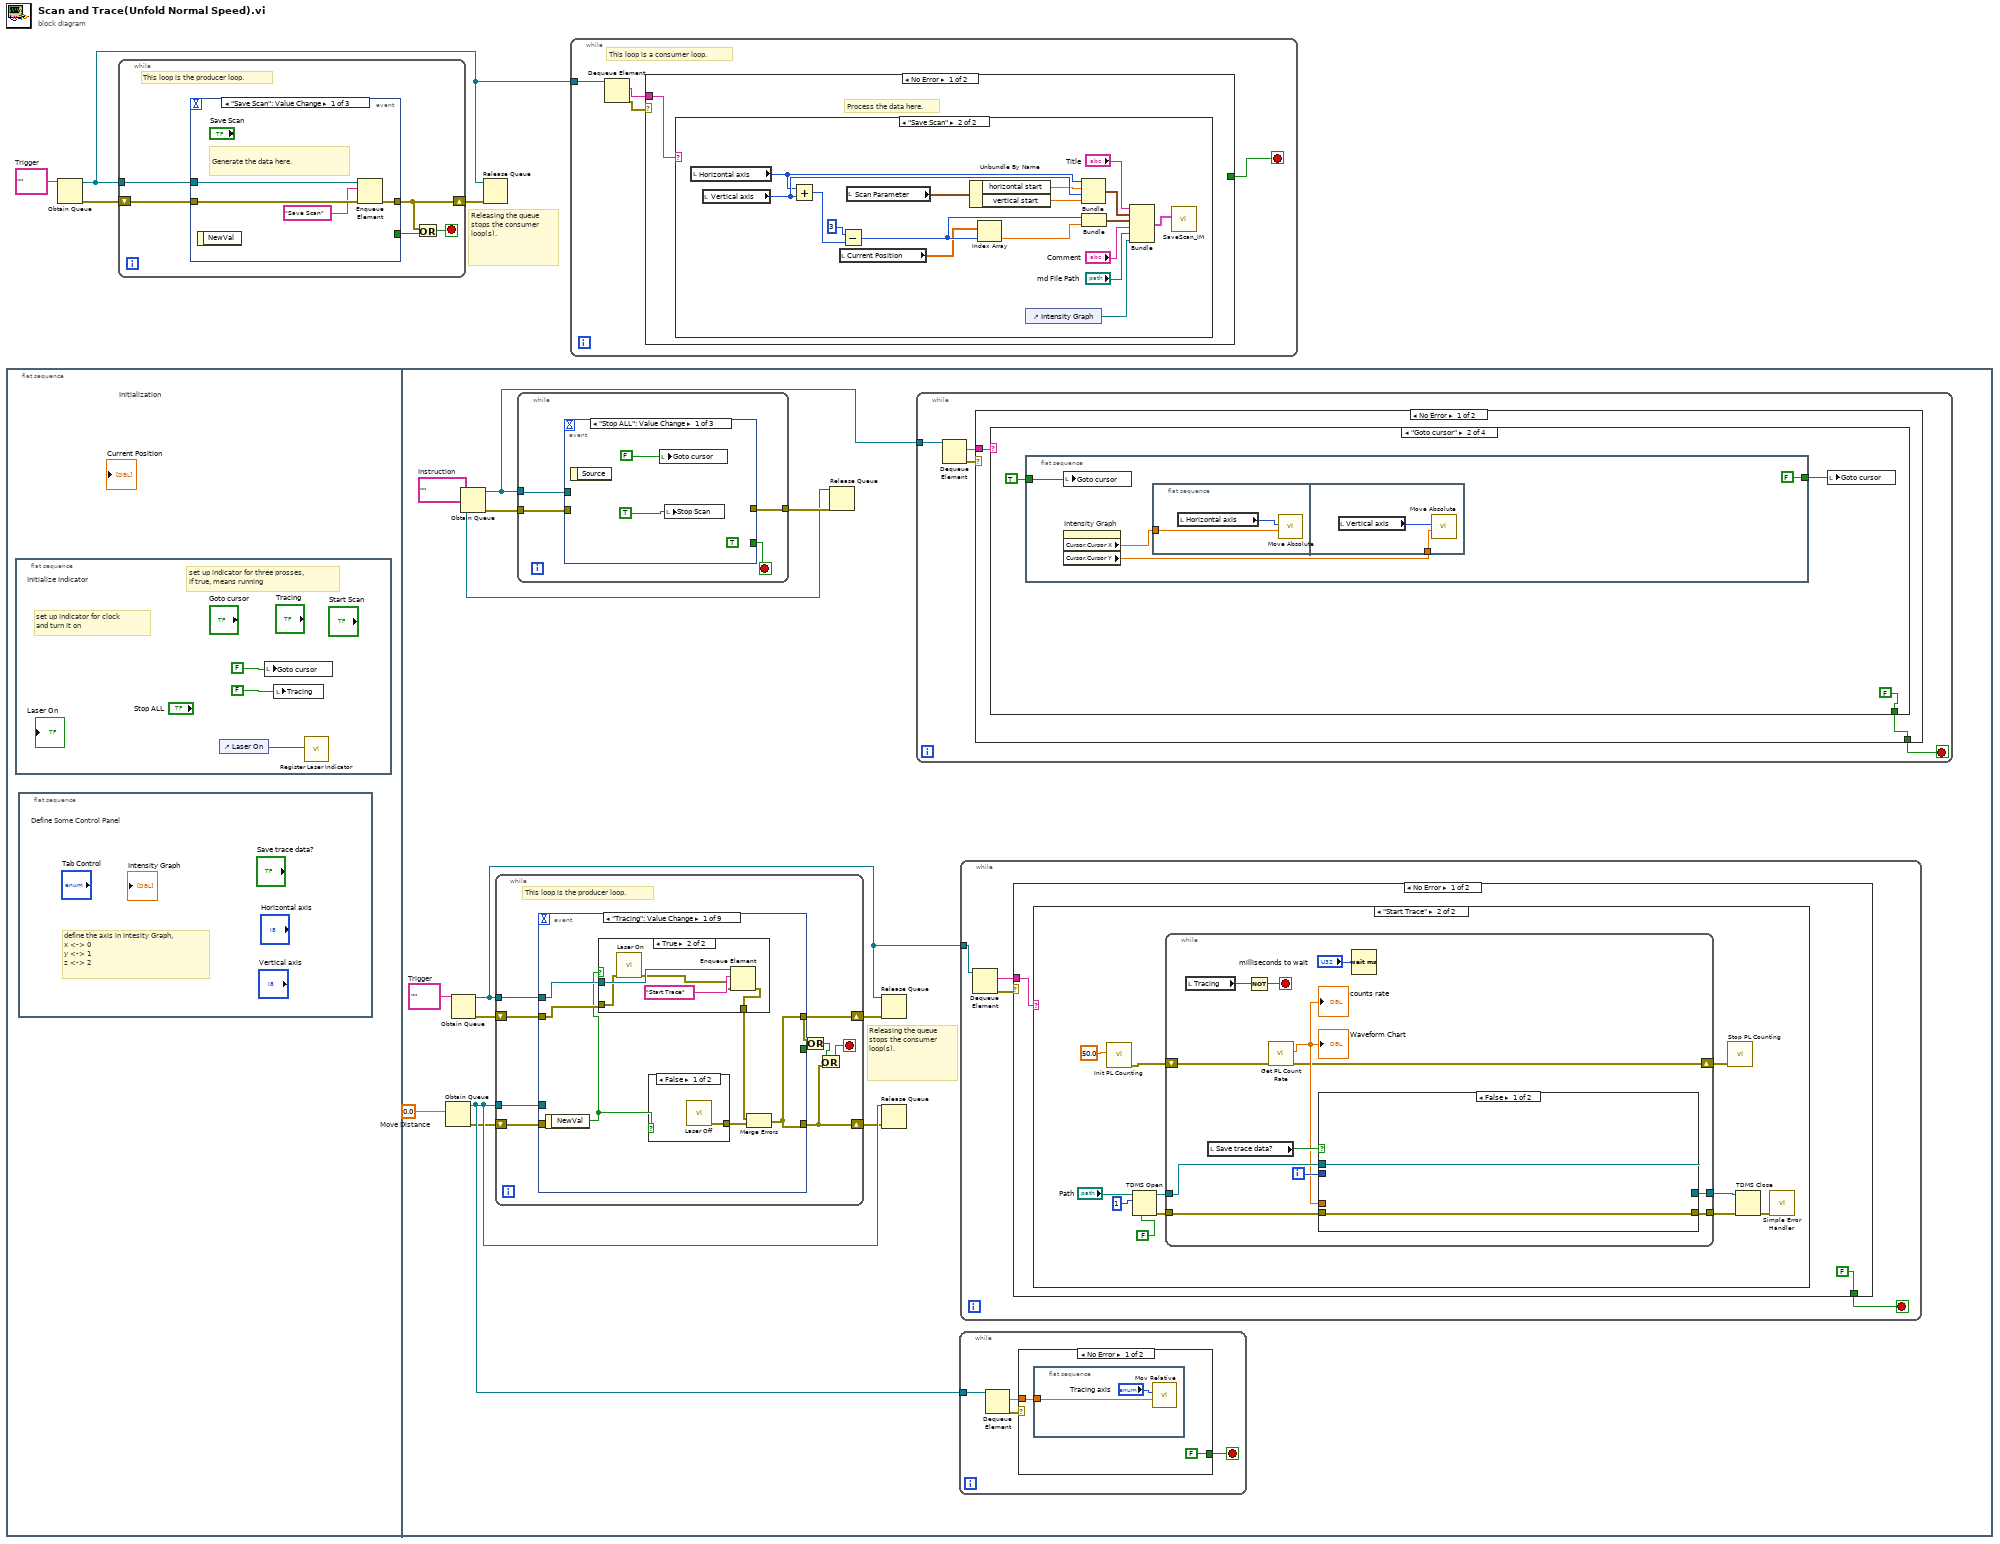
[diagram p0: block diagram]
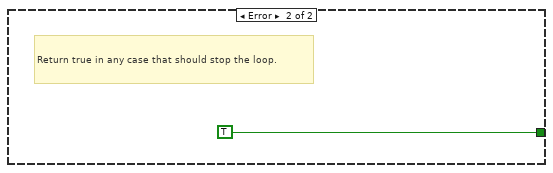
[diagram p3: hidden frame]
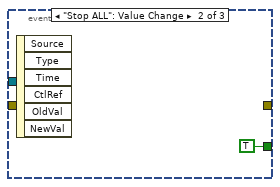
[diagram p4: hidden frame]
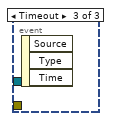
[diagram p5: hidden frame]
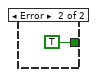
[diagram p6: hidden frame]
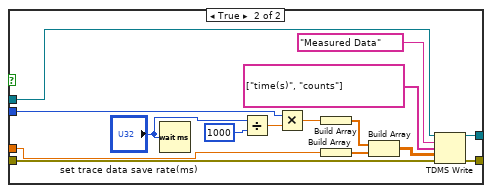
[diagram p8: hidden frame]
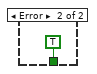
[diagram p9: hidden frame]
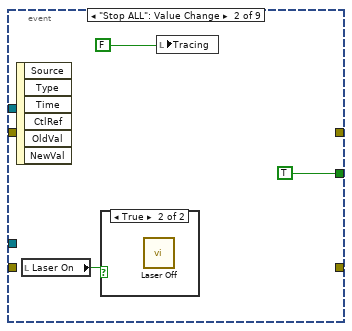
[diagram p12: hidden frame]
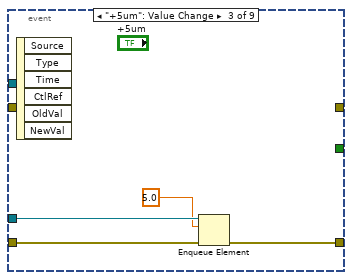
[diagram p14: hidden frame]
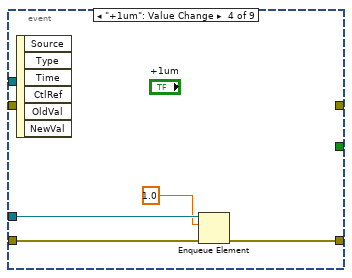
[diagram p15: hidden frame]
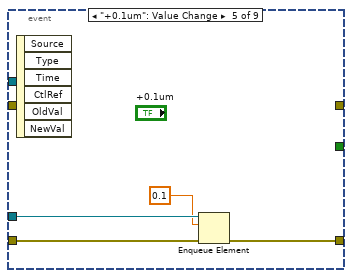
[diagram p16: hidden frame]
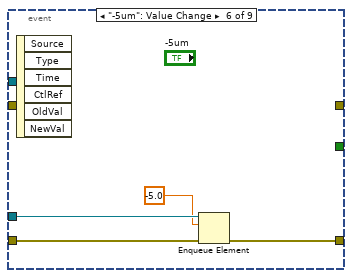
[diagram p17: hidden frame]
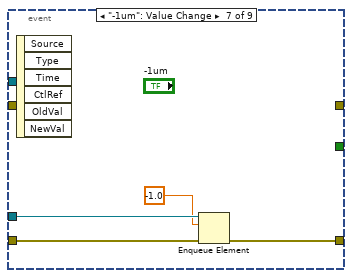
[diagram p18: hidden frame]
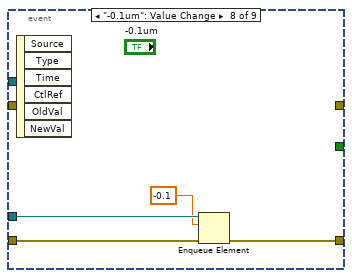
[diagram p19: hidden frame]
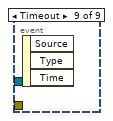
[diagram p20: hidden frame]
diagram:
  w2 = ""  # Trigger
  # "Releasing the queue stops the consumer loop(s)."
  n1 = flat-sequence {
    frame #0 {
      # "Initialization"
      n2 = flat-sequence {
        frame #0 {
          # "Initialize Indicator"
          # "set up indicator for clock \nand turn it on"
          # "set up indicator for three prosses,\nif true, means running"
          n3 = control-ref of="Laser On"() -> (w5:refnum<vi>)
          n4 = local write "Goto cursor"(FALSE) -> ()
          n5 = local write "Tracing"(FALSE) -> ()
          n6 = call "Register Laser Indicator.vi"("Laser Indicator Ref"=w5) -> ()  [unwired: 10 in, 1 out]
        }
      }
      n7 = flat-sequence {
        frame #0 {
          # "Define Some Control Panel"
          # "define the axis in Intesity Graph,\nx <-> 0\ny <-> 1\nz <-> 2"
        }
      }
    }
    frame #1 {
      w9 = 0.0  # Move Distance
      w8 = ""  # Trigger
      w19 = ""  # Instruction
      # "Releasing the queue stops the consumer loop(s)."
      n8 = Obtain Queue(element data type=w9) -> (queue out=w15:refnum<queue>, error out=w13:errorcluster)  [unwired: 4 in, 1 out]
      n9 = Obtain Queue(element data type=w8) -> (queue out=w12:refnum<queue>, error out=w10:errorcluster)  [unwired: 4 in, 1 out]
      n10 = Obtain Queue(element data type=w19) -> (queue out=w16:refnum<queue>, error out=w18:errorcluster)  [unwired: 4 in, 1 out]
      n11 = while {
        shift-right: [w81] -> w11
        shift-left: w10 -> [w83]
        tunnel: w12 -> [w84]
        shift-right: [w76] -> w14
        shift-left: w13 -> [w79]
        tunnel: w15 -> [w80]
        stop <- w77 stop-if-true
        # "This loop is the producer loop."
        n12 = event shown="[0] \"Tracing\": Value Change" {
          selector: _ -> [_ _ _ _ _ _ _ _ _]
          dyn-events: _ -> [_ _ _ _ _ _ _ _ _]
          timeout: _ -> [_ _ _ _ _ _ _ _ _]
          tunnel: w84 -> [w90 _ _ _ _ _ _ _ _]
          tunnel: w83 -> [w89 _ _ _ _ _ _ _ _]
          tunnel: [w87 _ _ _ _ _ _ _ _] -> w81
          tunnel: [_ TRUE ("stop") _ _ _ _ _ _ _] -> w82
          tunnel: w80 -> [_ _ w103 w107 w111 w115 w119 w123 _]
          tunnel: w79 -> [_ _ w102 w106 w110 w114 w118 w122 _]
          tunnel: [w87 _ w101 w105 w109 w113 w117 w121 _] -> w76
          event "Tracing": Value Change {
            n13 = event-data() -> ("NewVal"=w85:bool)  [unwired: 1 in]
            n14 = case shown="True" w85 {
              tunnel: w90 -> [_ w94]
              tunnel: w89 -> [_ w93]
              tunnel: [_ w91] -> w86
              frame False {
              }
              frame True {
                n15 = call "Laser On.vi"("error in"=w93) -> ("error out"=w92:errorcluster)  [unwired: 10 in]
                n16 = Enqueue Element(queue=w94, element="Start Trace", error in (no error)=w92) -> (error out=w91:errorcluster)  [unwired: 1 in, 2 out]
              }
            }
            n17 = case shown="False" w85 {
              tunnel: [w96 _] -> w88
              frame False {
                n18 = call "Laser Off.vi"() -> ("error out"=w96:errorcluster)  [unwired: 11 in]
              }
              frame True {
              }
            }
            n19 = Merge Errors(w86, w88) -> (w87:errorcluster)
          }
          event "Stop ALL": Value Change {
            n20 = event-data() -> ()  [unwired: 1 in, 6 out]
            n21 = local read "Laser On"() -> (w97:bool)
            n22 = case shown="True" w97 {
              frame False {
              }
              frame True {
                n23 = call "Laser Off.vi"() -> ()  [unwired: 11 in, 1 out]
              }
            }
            n24 = local write "Tracing"(FALSE ("Tracing")) -> ()
          }
          event "+5um": Value Change {
            n25 = event-data() -> ()  [unwired: 1 in, 6 out]
            n26 = Enqueue Element(queue=w103, element=5.0, error in (no error)=w102) -> (error out=w101:errorcluster)  [unwired: 1 in, 2 out]
          }
          event "+1um": Value Change {
            n27 = event-data() -> ()  [unwired: 1 in, 6 out]
            n28 = Enqueue Element(queue=w107, element=1.0, error in (no error)=w106) -> (error out=w105:errorcluster)  [unwired: 1 in, 2 out]
          }
          event "+0.1um": Value Change {
            n29 = event-data() -> ()  [unwired: 1 in, 6 out]
            n30 = Enqueue Element(queue=w111, element=0.1, error in (no error)=w110) -> (error out=w109:errorcluster)  [unwired: 1 in, 2 out]
          }
          event "-5um": Value Change {
            n31 = event-data() -> ()  [unwired: 1 in, 6 out]
            n32 = Enqueue Element(queue=w115, element=-5.0, error in (no error)=w114) -> (error out=w113:errorcluster)  [unwired: 1 in, 2 out]
          }
          event "-1um": Value Change {
            n33 = event-data() -> ()  [unwired: 1 in, 6 out]
            n34 = Enqueue Element(queue=w119, element=-1.0, error in (no error)=w118) -> (error out=w117:errorcluster)  [unwired: 1 in, 2 out]
          }
          event "-0.1um": Value Change {
            n35 = event-data() -> ()  [unwired: 1 in, 6 out]
            n36 = Enqueue Element(queue=w123, element=-0.1, error in (no error)=w122) -> (error out=w121:errorcluster)  [unwired: 1 in, 2 out]
          }
          event Timeout {
            n37 = event-data() -> ()  [unwired: 1 in, 3 out]
          }
        }
        n38 = Or(x=w81, y=w82) -> (x .or. y?=w78:bool)
        n39 = Or(x=w78, y=w76) -> (x .or. y?=w77:bool)
      }
      n40 = while {
        tunnel: w16 -> [w126]
        tunnel: w18 -> [w125]
        tunnel: [w124] -> w17
        stop <- w127 stop-if-true
        n41 = event shown="[0] \"Stop ALL\": Value Change" {
          selector: _ -> [_ _ _]
          dyn-events: _ -> [_ _ _]
          timeout: _ -> [_ _ _]
          tunnel: [TRUE FALSE FALSE] -> w127
          tunnel: w126 -> [_ w135 w144]
          tunnel: w125 -> [_ w134 w143]
          tunnel: [_ w133 w142] -> w124
          event "Stop ALL": Value Change {
            (unwired) TRUE
            n42 = event-data() -> ()  [unwired: 1 in, 1 out]
            n43 = local write "Goto cursor"(FALSE) -> ()
            n44 = local write "Stop Scan"(TRUE) -> ()
          }
          event "Start Scan": Value Change {
            (unwired) FALSE
            n45 = event-data() -> ("NewVal"=w131:bool)  [unwired: 1 in]
            n46 = case shown="True" w131 {
              tunnel: w135 -> [_ w140]
              tunnel: w134 -> [w136 w138]
              tunnel: [w136 w137] -> w133
              frame False {
              }
              frame True {
                n47 = Enqueue Element(queue=w140, element="Scan", error in (no error)=w138) -> (error out=w137:errorcluster)  [unwired: 1 in, 2 out]
              }
            }
          }
          event "go to crusor": Value Change {
            n48 = event-data() -> ()  [unwired: 1 in, 2 out]
            n49 = Enqueue Element(queue=w144, element="Goto cursor", error in (no error)=w143) -> (error out=w142:errorcluster)  [unwired: 1 in, 2 out]
          }
        }
      }
      n50 = Release Queue(queue=w16, error in (no error)=w17) -> ()  [unwired: 1 in, 3 out]
      n51 = Release Queue(queue=w12, error in (no error)=w11) -> ()  [unwired: 1 in, 3 out]
      n52 = Release Queue(queue=w15, error in (no error)=w14) -> ()  [unwired: 1 in, 3 out]
      n53 = while {
        tunnel: w16 -> [w149]
        stop <- w146 stop-if-true
        n54 = Dequeue Element(queue=w149) -> (element=w147:string, error out=w148:errorcluster)  [unwired: 2 in, 2 out]
        n55 = case shown="No Error" w148 {
          tunnel: w147 -> [w151 _]
          tunnel: [w150 TRUE] -> w146
          frame No Error {
            n56 = case shown="\"Goto cursor\"" w151 {
              tunnel: [FALSE FALSE TRUE FALSE] -> w150
              frame "Scan" {
                n57 = flat-sequence {
                  frame #0 {
                    n58 = local write "Stop Scan"(FALSE) -> ()
                  }
                  frame #1 {
                    n59 = local read "Horizontal axis"() -> (w160:i8)
                    n60 = local read "Vertical axis"() -> (w159:i8)
                    n61 = control-ref of="Current Position"() -> (w155:refnum<vi>)
                    n62 = control-ref of="Stop Scan"() -> (w154:refnum<vi>)
                    n63 = control-ref of="Intensity Graph"() -> (w156:refnum<vi>)
                    n64 = Bundle("Horizontal axis"=w160, "Vertical axis"=w159, "Scan Parameter"="Scan Parameter") -> (w157:T3)  [unwired: 1 in]
                    n65 = call "Scan.vi"(8:w155, "Intensity Graph Ref"=w156, "Stop Ref"=w154, "Scan parameter"=w157) -> ()  [unwired: 6 in, 2 out]
                  }
                  frame #2 {
                  }
                }
              }
              frame "Goto cursor" {
                n66 = flat-sequence {
                  tunnel: [FALSE] -> w163
                  tunnel: TRUE -> [w164]
                  frame #0 {
                    n67 = local write "Goto cursor"(w164) -> ()
                    n68 = property on="Intensity Graph" class="IntGraph (strict)"() -> ("Cursor.Cursor X"=w167:dbl, "Cursor.Cursor Y"=w166:dbl)  [unwired: 2 in, 2 out]
                    n69 = flat-sequence {
                      tunnel: w167 -> [w168]
                      tunnel: w166 -> [w171]
                      frame #0 {
                        n70 = local read "Horizontal axis"() -> (w169:i8)
                        n71 = call "Move Absolute.vi"("Goal Position"=w168, "Axis To Move"=w169) -> ()  [unwired: 8 in, 2 out]
                      }
                      frame #1 {
                        n72 = local read "Vertical axis"() -> (w170:i8)
                        n73 = call "Move Absolute.vi"("Goal Position"=w171, "Axis To Move"=w170) -> ()  [unwired: 8 in, 2 out]
                      }
                    }
                  }
                }
                n74 = local write "Goto cursor"(w163) -> ()
              }
              frame "Stop" {
              }
              frame "Invalid Message", Default {
              }
            }
          }
          frame Error {
          }
        }
      }
      n75 = while {
        tunnel: w15 -> [w23]
        stop <- w20 stop-if-true
        n76 = Dequeue Element(queue=w23) -> (element=w21:dbl, error out=w22:errorcluster)  [unwired: 2 in, 2 out]
        n77 = case shown="No Error" w22 {
          tunnel: w21 -> [w25 _]
          tunnel: [FALSE TRUE] -> w20
          frame No Error {
            n78 = flat-sequence {
              tunnel: w25 -> [w26]
              frame #0 {
                n79 = call "Mov Relative.vi"("Move Step"=w26, "Axis To Move"="Tracing axis") -> ()  [unwired: 8 in, 2 out]
              }
            }
          }
          frame Error {
          }
        }
      }
      n80 = while {
        tunnel: w12 -> [w32]
        stop <- w29 stop-if-true
        n81 = Dequeue Element(queue=w32) -> (element=w30:string, error out=w31:errorcluster)  [unwired: 2 in, 2 out]
        n82 = case shown="No Error" w31 {
          tunnel: w30 -> [w34 _]
          tunnel: [FALSE TRUE] -> w29
          frame No Error {
            n83 = case shown="\"Start Trace\"" w34 {
              frame "False", Default {
              }
              frame "Start Trace" {
                n84 = call "Init PL Counting.vi"("Sample Rate (Hz)"=50.0) -> ("error out"=w36:errorcluster)  [unwired: 10 in]
                n85 = TDMS Open(6:FALSE ("disable buffering (T)"), 10:1, 11:"Path") -> (0:w40:errorcluster, 3:w41:refnum<k34>)  [unwired: 4 in]
                n86 = while {
                  tunnel: w40 -> [w56]
                  tunnel: w41 -> [w55]
                  tunnel: [w53] -> w43
                  tunnel: [w52] -> w44
                  shift-right: [w46] -> w35
                  shift-left: w36 -> [w47]
                  i -> [w57]
                  stop <- w49 stop-if-true
                  n87 = local read "Tracing"() -> (w51:bool)
                  n88 = local read "Save trace data?"() -> (w54:bool)
                  n89 = Not(x=w51) -> (.not. x?=w49:bool)
                  n90 = call "Get PL Count Rate.vi"("error in (no error)"=w47) -> ("error out"=w46:errorcluster, "Count Rate"=w48:dbl)  [unwired: 8 in, 1 out]
                  "counts rate" <- w48
                  "Waveform Chart" <- w48
                  n91 = case shown="False" w54 {
                    tunnel: w55 -> [w59 w66]
                    tunnel: [w59 w65] -> w53
                    tunnel: w48 -> [_ w60]
                    tunnel: w56 -> [w58 w64]
                    tunnel: [w58 w63] -> w52
                    tunnel: w57 -> [_ w62]
                    frame False {
                    }
                    frame True {
                      n92 = Wait (ms)(milliseconds to wait="set trace data save rate(ms)") -> ()  [unwired: 1 out]
                      n93 = Divide(x="set trace data save rate(ms)", y=u32 1000) -> (x/y=w68:dbl)
                      n94 = Multiply(x=w62, y=w68) -> (x*y=w67:dbl)
                      n95 = Build Array(w67) -> (w72:dbl[])
                      n96 = Build Array(w60) -> (w71:dbl[])
                      n97 = Build Array(w72, w71) -> (w70:dbl[][])
                      n98 = TDMS Write(0:w66, 5:"Measured Data" ("group name"), 7:string[] ["time(s)", "counts"] ("channel names"), 9:w70, 11:w64) -> (4:w65:refnum<k34>, 15:w63:errorcluster)  [unwired: 1 in, 2 out]
                    }
                  }
                  n99 = Wait (ms)(milliseconds to wait="milliseconds to wait") -> ()  [unwired: 1 out]
                }
                n100 = call "Stop PL Counting.vi"("error in (no error)"=w35) -> ()  [unwired: 10 in, 1 out]
                n101 = TDMS Close(8:w44, 11:w43) -> (0:w42:errorcluster)  [unwired: 1 out]
                n102 = call <vilib>:"Simple Error Handler.vi"("error in (no error)"=w42) -> ()  [unwired: 1 in, 8 out]
              }
            }
          }
          frame Error {
          }
        }
      }
    }
  }
  n103 = Obtain Queue(element data type=w2) -> (queue out=w1:refnum<queue>, error out=w4:errorcluster)  [unwired: 4 in, 1 out]
  n104 = while {
    shift-right: [w175] -> w3
    shift-left: w4 -> [w178]
    tunnel: w1 -> [w179]
    stop <- w176 stop-if-true
    # "This loop is the producer loop."
    n105 = event shown="[0] \"Save Scan\": Value Change" {
      selector: _ -> [_ _ _]
      dyn-events: _ -> [_ _ _]
      timeout: _ -> [_ _ _]
      tunnel: w179 -> [w183 _ _]
      tunnel: w178 -> [w182 _ _]
      tunnel: [w181 _ _] -> w175
      tunnel: [_ TRUE ("stop") _] -> w177
      event "Save Scan": Value Change {
        # "Generate the data here."
        n106 = event-data() -> ()  [unwired: 1 in, 1 out]
        n107 = Enqueue Element(queue=w183, element="Save Scan", error in (no error)=w182) -> (error out=w181:errorcluster)  [unwired: 1 in, 2 out]
      }
      event "Stop ALL": Value Change {
        n108 = event-data() -> ()  [unwired: 1 in, 6 out]
      }
      event Timeout {
        n109 = event-data() -> ()  [unwired: 1 in, 3 out]
      }
    }
    n110 = Or(x=w175, y=w177) -> (x .or. y?=w176:bool)
  }
  n111 = Release Queue(queue=w1, error in (no error)=w3) -> ()  [unwired: 1 in, 3 out]
  n112 = while {
    tunnel: w1 -> [w188]
    stop <- w185 stop-if-true
    # "This loop is a consumer loop."
    n113 = Dequeue Element(queue=w188) -> (element=w186:string, error out=w187:errorcluster)  [unwired: 2 in, 2 out]
    n114 = case shown="No Error" w187 {
      tunnel: w186 -> [w189 _]
      tunnel: [_ TRUE] -> w185
      frame No Error {
        # "Process the data here."
        n115 = case shown="\"Save Scan\"" w189 {
          frame "False", Default {
          }
          frame "Save Scan" {
            n116 = local read "Horizontal axis"() -> (w196:i8)
            n117 = local read "Vertical axis"() -> (w197:i8)
            n118 = Add(x=w196, y=w197) -> (x+y=w195:i8)
            n119 = local read "Current Position"() -> (w198:dbl[])
            n120 = Subtract(x=3, y=w195) -> (x-y=w199:i32)
            n121 = local read "Scan Parameter"() -> (w192:T2)
            n122 = Unbundle By Name(w192) -> ("horizontal start"=w193:dbl, "vertical start"=w194:dbl)
            n123 = Index Array(array=w198, index=w199) -> (element=w200:dbl)
            n124 = control-ref of="Intensity Graph"() -> (w206:refnum<vi>)
            n125 = Bundle("Horizontal axis"=w196, "horizontal start"=w193, "Vertical axis"=w197, "vertical start"=w194) -> (w202:T4)  [unwired: 1 in]
            n126 = Bundle(w199, "position out"=w200) -> (w203:cluster{i32, "position out":dbl})  [unwired: 1 in]
            n127 = Bundle("Title"="Title", w202, w203, "Comment"="Comment", "md File Path"="md File Path", "Intensity Graph"=w206) -> (w190:T5)  [unwired: 1 in]
            n128 = call "SaveScan_IM.vi"("ScanSave Parameter"=w190) -> ()  [unwired: 10 in, 1 out]
          }
        }
      }
      frame Error {
        # "Return true in any case that should stop the loop."
      }
    }
  }
